vi "Generate Schema $defs From Path.vi"(8 "error in (no error)":errorcluster, 11 "ctl path":path) -> (0 "error out":errorcluster, 2 "Value":variant)   [LabVIEW 2019, in "JSON-Schema.lvlib"]
uses:
  JSON-Schema.lvlib
  <vilib>/Utility/Data Type/NI_Data Type.lvlib
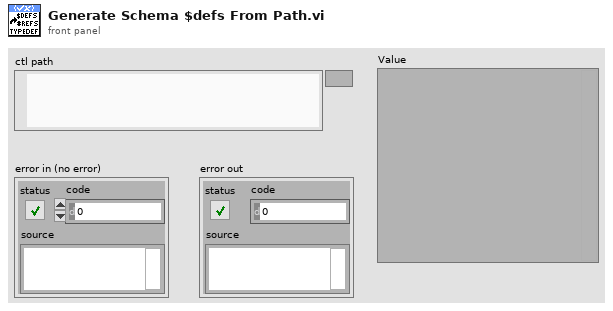
[diagram p1: front panel]
types:
  T1 = typedef "NI_Data Type.lvlib/Data Type.ctl" = enum8{"Invalid Type", "Void", "I8", "I16", "I32", "I64", "U8", "U16", "U32", "U64", "Single Float", "Double Float", "Extended Float", "Single Complex", "Double Complex", "Extended Complex", "Enum U8", "Enum U16", "Enum U32", "Enum U64", "Single Float With Unit", "Double Float With Unit", "Extended Float With Unit", "Single Complex with Unit", "Double Complex with Unit", "Extended Complex with Unit", "Boolean", "String", "Path", "Picture", "Tag", "Array", "Cluster", "Variant", "LV Variant", "Waveform", "Timestamp", "Digital Waveform", "Digital Data", "ExpressData", "Refnum", "External Data", "VI", "Poly VI", "LabVIEW Class Instance", "Fixed Point", "Set Collection", "Map Collection"}
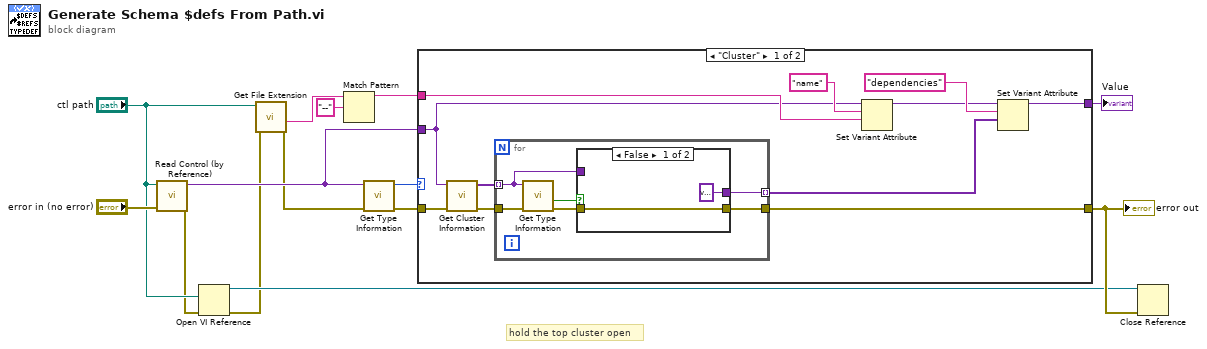
[diagram p0: block diagram]
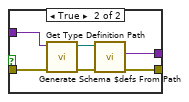
[diagram p2: hidden frame]
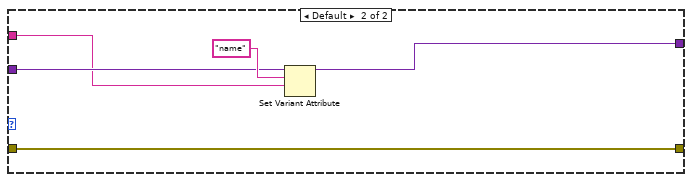
[diagram p3: hidden frame]
diagram:
  # "hold the top cluster open"
  n1 = call "Read Control (by Reference).vi"("error in (no error)"="error in (no error)", "ctl path"="ctl path") -> ("error out"=w5:errorcluster, "Value"=w14:variant)  [unwired: 7 in, 1 out]
  n2 = Open VI Reference(vi path="ctl path", error in (no error)=w5) -> (vi reference=w3:refnum<vi>, error out=w2:errorcluster)  [unwired: 4 in]
  n3 = call <vilib>:"Get File Extension.vi"("error in (no error)"=w2, "file"="ctl path") -> ("error out"=w10:errorcluster, "filename without extension"=w8:string)  [unwired: 5 in, 3 out]
  n4 = Match Pattern(string=w8, regular expression="--") -> (before substring=w7:string)  [unwired: 1 in, 3 out]
  n5 = call <vilib>:"Get Type Information.vi"("error in (no error)"=w10, "variant"=w14) -> ("error out"=w11:errorcluster, "type"=w12:T1)  [unwired: 5 in, 3 out]
  n6 = case shown="\"Cluster\"" w12 {
    tunnel: w14 -> [w16 w42]
    tunnel: w11 -> [w23 w44]
    tunnel: [w22 w44] -> w4
    tunnel: w7 -> [w18 w41]
    tunnel: [w15 w40] -> w1
    frame "Cluster" {
      n7 = call <vilib>:"Get Cluster Information.vi"("error in (no error)"=w23, "variant"=w16) -> ("error out"=w24:errorcluster, "cluster elements"=w25:variant[])  [unwired: 8 in]
      n8 = for {
        tunnel: w25 -> [w29] mode=indexing
        tunnel: w24 -> [w31]
        tunnel: [w27] -> w22
        tunnel: [w26] -> w21 mode=indexing
        n9 = call <vilib>:"Get Type Information.vi"("error in (no error)"=w31, "variant"=w29) -> ("error out"=w28:errorcluster, "type definition"=w30:bool)  [unwired: 5 in, 3 out]
        n10 = case shown="False" w30 {
          tunnel: w29 -> [_ w38]
          tunnel: w28 -> [w33 w39]
          tunnel: [w33 w35] -> w27
          tunnel: [variant ("Value") w34] -> w26
          frame False {
          }
          frame True {
            n11 = call <vilib>:"Get Type Definition Path.vi"("error in (no error)"=w39, "variant"=w38) -> ("error out"=w37:errorcluster, "type definition path"=w36:path)  [unwired: 8 in]
            n12 = call "Generate Schema $defs From Path.vi"("error in (no error)"=w37, "ctl path"=w36) -> ("error out"=w35:errorcluster, "Value"=w34:variant)  [unwired: 8 in]
          }
        }
      }
      n13 = Set Variant Attribute(Variant=w16, name="name", value=w18) -> (Variant out=w17:variant)  [unwired: 1 in, 2 out]
      n14 = Set Variant Attribute(Variant=w17, name="dependencies", value=w21) -> (Variant out=w15:variant)  [unwired: 1 in, 2 out]
    }
    frame Default {
      n15 = Set Variant Attribute(Variant=w42, name="name", value=w41) -> (Variant out=w40:variant)  [unwired: 1 in, 2 out]
    }
  }
  "error out" <- w4
  "Value" <- w1
  n16 = Close Reference(reference=w3, error in (no error)=w4) -> ()  [unwired: 1 out]
